vi "良率计算VI.vi"(10 "M4A数据":string[](array[string])=["1", "NG", "dd", "dd", "f", "g"], 11 "良率结算结果":string[](array[string])) -> (3 "判断结果输出":string[](array[string]))   [LabVIEW 2011]
panel:
  out "M4 ThroughtRate":string
  out "M4 CumRetestYield":string
  out "M4 ReTest":string
  out "M4 Failing Rate":string
  out "NG":string
  out "Pass":string
  out "NG":string
  out "Pass":string
  out "总数":string
  out "总数":string
  out "M4 FPYR":string
  out "M4 Result":string
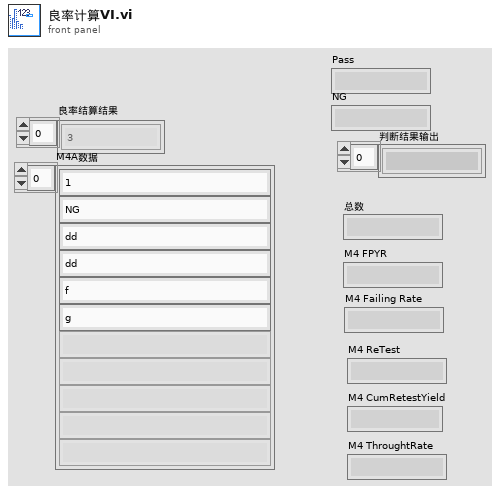
[diagram p1: front panel]
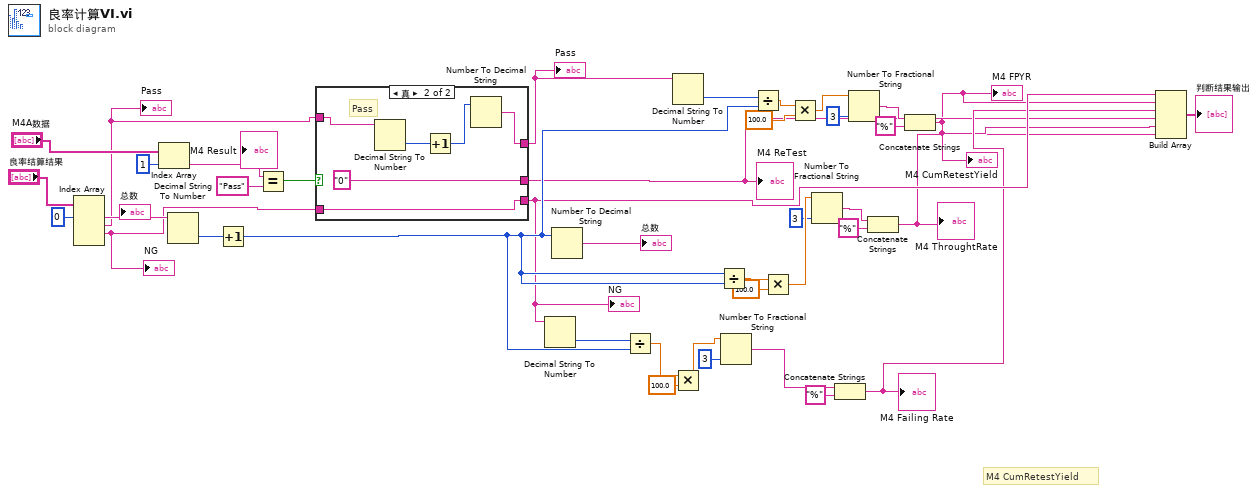
[diagram p0: block diagram]
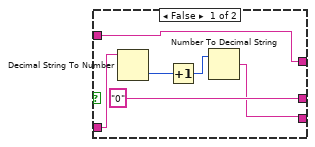
[diagram p2: hidden frame]
diagram:
  # "M4 CumRetestYield"
  n1 = Index Array(array="良率结算结果", index #1=0 ("索引")) -> (element #1=w33:string, element #2=w30:string, element #3=w29:string)  [unwired: 3 in, 1 out]
  "总数" <- w33
  "Pass" <- w30
  "NG" <- w29
  n2 = Index Array(array="M4A数据", index=1 ("索引")) -> (element=w38:string)
  "M4 Result" <- w38
  n3 = Decimal String To Number(string=w33) -> (number=w32:i32)  [unwired: 2 in, 1 out]
  n4 = Increment(x=w32) -> (x+1=w23:i32)
  n5 = Equal?(x=w38, y="Pass") -> (x = y?=w36:bool)
  n6 = case shown="真" w36 {
    tunnel: ["0" "0"] -> w4
    tunnel: w30 -> [w42 w50]
    tunnel: w29 -> [w44 w47]
    tunnel: [w42 w48] -> w26
    tunnel: [w41 w47] -> w6
    frame False {
      n7 = Decimal String To Number(string=w44) -> (number=w45:i32)  [unwired: 2 in, 1 out]
      n8 = Increment(x=w45) -> (x+1=w43:i32)
      n9 = Number To Decimal String(number=w43) -> (decimal integer string=w41:string)  [unwired: 1 in]
    }
    frame True {
      # "Pass"
      n10 = Decimal String To Number(string=w50) -> (number=w51:i32)  [unwired: 2 in, 1 out]
      n11 = Increment(x=w51) -> (x+1=w49:i32)
      n12 = Number To Decimal String(number=w49) -> (decimal integer string=w48:string)  [unwired: 1 in]
    }
  }
  "Pass" <- w26
  "NG" <- w6
  "M4 ReTest" <- w4
  n13 = Decimal String To Number(string=w6) -> (number=w28:i32)  [unwired: 2 in, 1 out]
  n14 = Number To Decimal String(number=w23) -> (decimal integer string=→"总数":string)  [unwired: 1 in]
  n15 = Divide(x=w28, y=w23) -> (x/y=w8:dbl)
  n16 = Decimal String To Number(string=w26) -> (number=w27:i32)  [unwired: 2 in, 1 out]
  n17 = Multiply(x=w8, y=100.0) -> (x*y=w7:dbl)
  n18 = Divide(x=w23, y=w23) -> (x/y=w22:dbl)
  n19 = Number To Fractional String(number=w7, precision (6)=i16 3 ("精度(6)")) -> (F-format string=w16:string)  [unwired: 2 in]
  n20 = Divide(x=w27, y=w23) -> (x/y=w12:dbl)
  n21 = Multiply(x=w22, y=100.0) -> (x*y=w18:dbl)
  n22 = Multiply(x=w12, y=100.0) -> (x*y=w10:dbl)
  n23 = Number To Fractional String(number=w18, precision (6)=i16 3 ("精度(6)")) -> (F-format string=w19:string)  [unwired: 2 in]
  n24 = Concatenate Strings(w16, "%" ("字符串")) -> (w5:string)
  "M4 Failing Rate" <- w5
  n25 = Number To Fractional String(number=w10, precision (6)=i16 3 ("精度(6)")) -> (F-format string=w25:string)  [unwired: 2 in]
  n26 = Concatenate Strings(w19, "%" ("字符串")) -> (w2:string)
  "M4 ThroughtRate" <- w2
  n27 = Concatenate Strings(w25, "%" ("字符串")) -> (w3:string)
  "M4 FPYR" <- w3
  "M4 CumRetestYield" <- w3
  n28 = Build Array(w6, w3, w5, w4, w3, w2) -> (→"判断结果输出":string[])
